vi "Output_SM.vi"(0 "SM Private Data in":refnum<class "Inspection Statemachine.lvclass">, 5 "Output Cluster":T1={"RackID"=0, "Trigger Light Camera Sequence"={"Light Sequence Trigger"="", "Status"="", "Mode"=""}, "Result Cluster"={"RackID"=0, "MeasurementValuesArray "=[], "ImagesArray"=[], "ResultPF"=FALSE, "ProductionCountDetails"={"TotalFail"=0, "TotalPass"=0, "TotalCount"=0}, "ReelCountDetails"={"ReelFail"=0, "ReelPass"=0, "ReelCount"=0}, "ControlPFArray"=[], "SpecificationPFArray"=[], "SpecificationFail"=FALSE, "ReelNumber"=0, "Status"=""}, "Analytics VI refnum"=refnum, "Statistical parameters "=[], "Sensor Name"="", "Camera Name"="", "PopupInput"={"Pop-up Type"=enum."Open Logo Display", "Title"="", "Message"="", "Button 1 Text"="", "Button 2 Text"="", "Show Close? T/F"=FALSE, "Title Blink? T/F"=FALSE, "Title Blink Colour"=0}, "PartInfo"={"PartName"="", "NumberOfRacks"=0, "TotalCount"=0, "ReelCount"=0, "OperatorName"="", "StampingMachineID"=0, "RackID"=0, "Reinitialize"=FALSE, "MeasurementNamesArray"=[], "MeasurementIDArray"=[], "SpecValuesArray"=[], "CameraNamesArray"=[]}, "StateMsgToMI"="", "InspectionStatusToMI"="", "StateMsgToRC"="", "StateMsgToUI"="", "StateMsgToDL"="", "StateMsgToAN"="", "StateMsgToSM"="", "EventData"={"EventName"="", "EventReason"=""}, "CameraOpticsDiagnosticsResult"={"LightCameraName"="", "DiagnosedImage"=refnum, "DustPercentage"=0.0, "Result"=TRUE}, "AllPartInfo"=[{"PartName"="", "NumberOfRacks"=0, "MeasurementIDsArray"=[], "MeasurementNamesArray"=[], "SpecValuesArray"=[]}], "SystemParameters"={"SystemName"="", "SystemID"="", "CustomerDetails"={"CustomerName"="", "CustomerId"="", "Location"="", "NumberOfShifts"=0.0, "ShiftDetails"=[]}, "InstallationDate"="", "NextServiceDate"="", "NumberOfRacks"=0, "TotalNumberOfCameras"=0, "SoftwareFeatures"={"HardwareEmulated"=FALSE, "PowerOnSelfTest"=FALSE, "DiagnosticsEnable"=FALSE, "AnalyticsEnable"=FALSE, "DefectTrackingEnable"=FALSE, "AutomaticGuideMovement"=FALSE, "DoorPokayokeEnable"=FALSE, "FailCountDisplayEnable"=FALSE, "FailCountReversalEnable"=FALSE, "DataLoggingEnable"=FALSE, "PauseOnReelCountFinish"=FALSE, "StopOnTotalCountFinish"=FALSE, "IoTEnable"=FALSE, "ReportEnable"=FALSE, "DebugLevel"=0.0, "PowerOnSelfTestFeatures"={"TimingUnit"=FALSE, "MachinePowerStatusCheck"=FALSE, "GuideMotor"=FALSE, "CameraOptics"=FALSE, "MasterSample"=FALSE}, "DiagnosticsFeatures"={"TimingUnit"=FALSE, "GuideMotor"=FALSE, "CameraOptics"=FALSE, "ReelerMotor"=FALSE, "HardwareButtons"=FALSE, "Sensors"=FALSE, "TowerLamp"=FALSE, "MasterSample"=FALSE}, "UserInterface"={"DynamicImageHandlingEnable"=FALSE, "DoorPokaYokeButtonVisible"=FALSE, "FailCountDisplayButtonVisible"=FALSE, "FailCountReversalButtonVisible"=FALSE}, "PopupOptions"={"ReasonForPause"=FALSE, "ReasonForFail"=FALSE, "ReasonForStop"=FALSE, "CpCpkOnReelFinish"=FALSE}, "DataloggingFeatures"={"EventData"=FALSE, "MeasurementData"=FALSE, "StatisticalData"=FALSE, "ReelData"=FALSE, "FailedMeasurementData"=FALSE, "FailedImages"=FALSE}, "IoT"={"SMSAlertEnable"=FALSE, "EmailAlertEnable"=FALSE}}}, "PartsConfigured"=[], "CameraSequenceList"=[], "SensorList"=[], "MasterSampleMessages"={"MasterSampleMessage"="", "PartMessage"=""}, "SensorDiagnosticsResult"={"Image Array"=[], "ImageCount"=0}, "IgnoredCountDetails"={"ReelCount"=0, "TotalCount"=0}, "MachineStatusToDL"="", "MasterSamplePartName"=""}, 7 "Receiver Name":string(combo), 9 "State":string, 11 "error in (no error)":errorcluster) -> (4 "SM Private Data out":refnum<class "Inspection Statemachine.lvclass">, 15 "error out":errorcluster)   [LabVIEW 2019, in "Inspection Statemachine.lvclass"]
uses:
  Inspection Statemachine.lvclass
  Rack Controller/Rack Controller Messages/RackId_RC Msg/Rack ID_RC Msg.lvclass
  Machine Interface/Machine Interface Messages/State Message from Inspection StateMachine Msg/State Message from Inspection StateMachine Msg_MI.lvclass
  Machine Interface/Machine Interface Messages/Trigger Light Camera Sequence Msg/Trigger Light Camera Sequence Msg_MI.lvclass
  Machine Interface/Machine Interface Messages/Enable and Power On sensor Msg/Enable and Power On Sensor_MI Msg.lvclass
  Machine Interface/Machine Interface Messages/Part Name from Inspection Statemachine Msg/Part Name from Inspection Statemachine Msg_MI.lvclass
  Machine Interface/Machine Interface Messages/Inspection Status Msg/Inspection Status Msg_MI.lvclass
  Rack Controller/Rack Controller Messages/StateMessage_RC Msg/State Message_RC Msg.lvclass
  Rack Controller/Rack Controller Messages/CameraOpticsDiagnostics_RC Msg/Camera Optics Diagnostics_RC Msg.lvclass
  Rack Controller/Rack Controller Messages/Selected Part Info_RC Msg/Selected Part Info_RC Msg.lvclass
  <vilib>/ActorFramework/Actor/Actor.lvclass
  <vilib>/ActorFramework/Message Enqueuer/Message Enqueuer.lvclass
  User Interface/User Interface Messages/User Interface messages/Pre-select init_UI Msg/SystemInfo_UI.lvclass
  User Interface/User Interface Actor/Type Definitions/JSON Read/Data initialization.ctl
  User Interface/User Interface Actor/ZenGage v3.0 UI.lvclass
  User Interface/User Interface Messages/User Interface messages/AN_Get analytics VI ref_UI Msg/GetAnalyticsVI_UI.lvclass
  DataLogger/DataLogger Messages/Part based Initialization_DL Msg/Part based Initialization_DL Msg.lvclass
  DataLogger/DataLogger Messages/Reel Info_DL Msg/Reel Info_DL Msg.lvclass
  DataLogger/DataLogger Messages/Event Info_DL Msg/Event Info_DL Msg.lvclass
  <vilib>/vision/Image Controls.llb/IMAQ Image.ctl
  DataLogger/DataLogger Messages/Statistical Info_DL Msg/Statistical Info_DL Msg.lvclass
  DataLogger/DataLogger Messages/Batch Info_DL Msg/Batch Info_DL Msg.lvclass
  DataLogger/DataLogger Messages/State Message_DL Msg/State Message_DL Msg.lvclass
  DataLogger/DataLogger Messages/AllPartInitialization_DL Msg/AllPartInitialization_DL Msg.lvclass
  DataLogger/DataLogger Messages/System Info_DL Msg/System Info_DL Msg.lvclass
  User Interface/User Interface Messages/User Interface messages/Display Popup Msg/DisplayPopup_UI.lvclass
  User Interface/User Interface Messages/User Interface messages/Call function_UI Msg/ButtonPress_UI.lvclass
  User Interface/User Interface Messages/User Interface messages/Post-select init_UI Msg/PartInfo_UI.lvclass
  User Interface/User Interface Actor/Type Definitions/JSON Read/Post select init.ctl
  User Interface/User Interface Messages/User Interface messages/RC_Result Cluster User Event_UI Msg/DisplayResult_UI Msg.lvclass
  User Interface/User Interface Actor/Type Definitions/Inspection/Result Cluster.ctl
  User Interface/User Interface Messages/User Interface messages/AskEventReason_UI Msg/AskEventReason_UI Msg.lvclass
  ZenAnalytics/Zen Analytics Messages/InterDataCommunication_ZA Msg/InterDataCommunication_ZA Msg.lvclass
  User Interface/User Interface Messages/User Interface messages/Display CpCpk data_UI Msg/Display CpCpk data_UI Msg.lvclass
  Common/Controls/Camera Optics Diagnostics.ctl
  User Interface/User Interface Messages/User Interface messages/Display master sample messages_UI Msg/DisplayMasterSampleMessages_UI Msg.lvclass
  User Interface/User Interface Messages/User Interface messages/CC_Sensor Trigger_UI Msg/TriggerSensorDiagnostics_UI.lvclass
  User Interface/User Interface Messages/User Interface messages/CC_Optics User Event_UI Msg/OpticsDiagnostics_UI.lvclass
  User Interface/User Interface Actor/Type Definitions/User Events UI/Optics diagnostics cluster.ctl
  Inspection Statemachine Messages/ButtonPressed_SM Msg/ButtonPressed_SM Msg.lvclass
  Inspection Statemachine Messages/DiagnosticsResult_SM Msg/DiagnosticsResult_SM Msg.lvclass
  Common/Controls/Diagnostics Result.ctl
  Rack Controller/Rack Controller Messages/IgnoredFailCountDetails_RC Msg/IgnoredFailCountDetails_RC Msg.lvclass
  DataLogger/DataLogger Messages/Measurement Info_DL Msg/Measurement Info_DL Msg.lvclass
  DataLogger/DataLogger Messages/Failure Info_DL Msg/Failure Info_DL Msg.lvclass
  DataLogger/DataLogger Messages/Machine Status_DL Msg/Machine Status_DL Msg.lvclass
  DataLogger/DataLogger Messages/MasterSample Info_DL Msg/MasterSample Info_DL Msg.lvclass
  C:/Program Files/National Instruments/LabVIEW 2019/vi.lib/ActorFramework/Actor/Actor.lvclass
  Controls/Result Cluster_SM.ctl
  Common/Controls/Pop-up Input.ctl
  Controls/Output Cluster_SM.ctl
  Common/Controls/Camera Optics Diagnostics Result.ctl
  Common/Controls/AllPartInfo.ctl
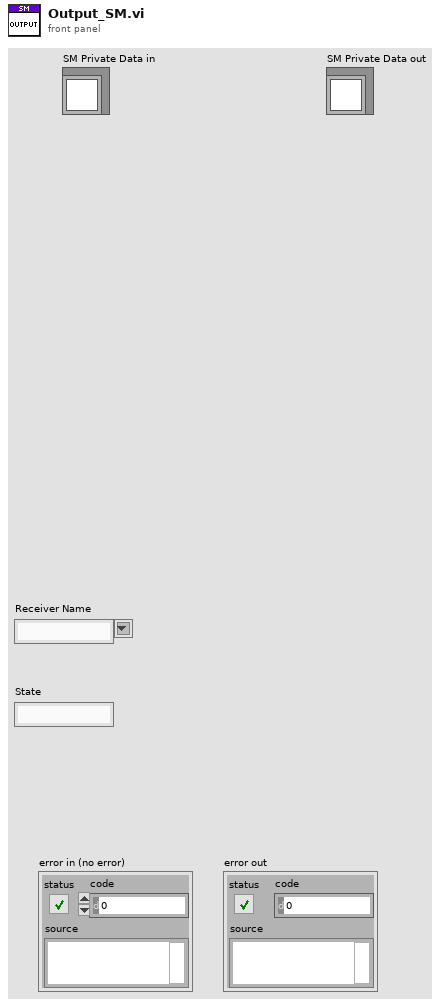
[diagram p1: front panel]
types:
  T1 = typedef "Inspection Statemachine.lvclass/Output Cluster_SM.ctl" = cluster{"RackID":u8, "Trigger Light Camera Sequence":cluster{"Light Sequence Trigger":string, "Status":string, "Mode":string}, "Result Cluster":T2, "Analytics VI refnum":refnum<vi>, "Statistical parameters ":string[][], "Sensor Name":string, "Camera Name":string, "PopupInput":T4, "PartInfo":cluster{"PartName":string, "NumberOfRacks":u8, "TotalCount":u64, "ReelCount":u64, "OperatorName":string, "StampingMachineID":u32, "RackID":u8, "Reinitialize":bool, "MeasurementNamesArray":string[], "MeasurementIDArray":u16[], "SpecValuesArray":cluster{"LCL":dbl, "UCL":dbl, "LSL":dbl, "USL":dbl, "Nominal Value":dbl}[], "CameraNamesArray":string[]}, "StateMsgToMI":string, "InspectionStatusToMI":string, "StateMsgToRC":string, "StateMsgToUI":string, "StateMsgToDL":string, "StateMsgToAN":string, "StateMsgToSM":string, "EventData":cluster{"EventName":string, "EventReason":string}, "CameraOpticsDiagnosticsResult":T5, "AllPartInfo":T6, "SystemParameters":cluster{"SystemName":string, "SystemID":string, "CustomerDetails":cluster{"CustomerName":string, "CustomerId":string, "Location":string, "NumberOfShifts":dbl, "ShiftDetails":cluster{"Name":string, "Timing":string}[]}, "InstallationDate":string, "NextServiceDate":string, "NumberOfRacks":u8, "TotalNumberOfCameras":u8, "SoftwareFeatures":cluster{"HardwareEmulated":bool, "PowerOnSelfTest":bool, "DiagnosticsEnable":bool, "AnalyticsEnable":bool, "DefectTrackingEnable":bool, "AutomaticGuideMovement":bool, "DoorPokayokeEnable":bool, "FailCountDisplayEnable":bool, "FailCountReversalEnable":bool, "DataLoggingEnable":bool, "PauseOnReelCountFinish":bool, "StopOnTotalCountFinish":bool, "IoTEnable":bool, "ReportEnable":bool, "DebugLevel":dbl, "PowerOnSelfTestFeatures":cluster{"TimingUnit":bool, "MachinePowerStatusCheck":bool, "GuideMotor":bool, "CameraOptics":bool, "MasterSample":bool}, "DiagnosticsFeatures":cluster{"TimingUnit":bool, "GuideMotor":bool, "CameraOptics":bool, "ReelerMotor":bool, "HardwareButtons":bool, "Sensors":bool, "TowerLamp":bool, "MasterSample":bool}, "UserInterface":cluster{"DynamicImageHandlingEnable":bool, "DoorPokaYokeButtonVisible":bool, "FailCountDisplayButtonVisible":bool, "FailCountReversalButtonVisible":bool}, "PopupOptions":cluster{"ReasonForPause":bool, "ReasonForFail":bool, "ReasonForStop":bool, "CpCpkOnReelFinish":bool}, "DataloggingFeatures":cluster{"EventData":bool, "MeasurementData":bool, "StatisticalData":bool, "ReelData":bool, "FailedMeasurementData":bool, "FailedImages":bool}, "IoT":cluster{"SMSAlertEnable":bool, "EmailAlertEnable":bool}}}, "PartsConfigured":cluster{"Name":string, "NumberOfRack":u8}[], "CameraSequenceList":cluster{"Name":string, "RackID":u8}[], "SensorList":cluster{"Name":string, "RackID":u8}[], "MasterSampleMessages":cluster{"MasterSampleMessage":string, "PartMessage":string}, "SensorDiagnosticsResult":cluster{"Image Array":T3[], "ImageCount":u64}, "IgnoredCountDetails":cluster{"ReelCount":u64, "TotalCount":u64}, "MachineStatusToDL":string, "MasterSamplePartName":string}
  T2 = typedef "Inspection Statemachine.lvclass/Result Cluster_SM.ctl" = cluster{"RackID":u8, "MeasurementValuesArray ":dbl[], "ImagesArray":T3[], "ResultPF":bool, "ProductionCountDetails":cluster{"TotalFail":u64, "TotalPass":u64, "TotalCount":u64}, "ReelCountDetails":cluster{"ReelFail":u64, "ReelPass":u64, "ReelCount":u64}, "ControlPFArray":bool[], "SpecificationPFArray":bool[], "SpecificationFail":bool, "ReelNumber":u64, "Status":string}
  T3 = typedef "IMAQ Image.ctl" = refnum<image>
  T4 = typedef "Pop-up Input.ctl" = cluster{"Pop-up Type":enum16{"Open Logo Display", "Close Logo Display", "Open Loading Bar", "Close Loading Bar", "Open Alert Display", "Close Alert Display", "One button dialog box", "Two button dialog box", "User Authentication"}, "Title":string, "Message":string, "Button 1 Text":string, "Button 2 Text":string, "Show Close? T/F":bool, "Title Blink? T/F":bool, "Title Blink Colour":u32}
  T5 = typedef "Camera Optics Diagnostics Result.ctl" = cluster{"LightCameraName":string, "DiagnosedImage":T3, "DustPercentage":dbl, "Result":bool}
  T6 = typedef "AllPartInfo.ctl" = cluster{"PartName":string, "NumberOfRacks":u8, "MeasurementIDsArray":u16[], "MeasurementNamesArray":string[], "SpecValuesArray":cluster{"LCL":dbl, "UCL":dbl, "LSL":dbl, "USL":dbl, "NominalValue":dbl}[]}[]
  T7 = typedef "Diagnostics Result.ctl" = cluster{"Result":bool, "StateMessage":string}
  T8 = typedef "Camera Optics Diagnostics.ctl" = cluster{"Light Camera Name":string, " State":string}
  T9 = cluster{"Master sample message":string, "Part message":string}
  T10 = typedef "ZenGage v3.0 UI.lvclass/Post select init.ctl" = cluster{"PartName":string, "RackId":u8, "ReInitialize":bool, "MeasurementNames":string[], "SpecValues":cluster{"LCL":dbl, "UCL":dbl, "LSL":dbl, "USL":dbl, "NominalValue":dbl}[], "CameraNames":string[]}
  T11 = typedef "ZenGage v3.0 UI.lvclass/Data initialization.ctl" = cluster{"DiagnosticsFeatures":cluster{"ArduinoDiagnostics":bool, "MotorDiagnostics":bool, "CameraOpticsDiagnostics":bool, "ReelerMotor":bool, "TowerLampDiagnostics":bool, "HardwareButtonDiagnostics":bool, "TriggerSensor":bool, "MasterSampleDiagnostics":bool}, "UserInterfaceButtonVisibilty":cluster{"Door Poka Yoke":bool, "DynamicImageHandlingEnable":bool, "FailCountDisplayButtonVisible":bool, "FailCountReversalButtonVisible":bool}, "Analytics enabled":bool, "Parts List":cluster{"Part name":string, "NumberOfRacks":u8}[]}
  T12 = cluster{"Reel Count":dbl, "Reel Pass":dbl, "Reel Fail":dbl}
  T13 = cluster{"Total Count":dbl, "Total Pass":dbl, "Total Fail":dbl}
  T14 = typedef "ZenGage v3.0 UI.lvclass/Result Cluster.ctl" = cluster{"Rack Id":u64, "Measurement Values Array ":dbl[], "Images_Array_in":T3[], "ResultPF":bool, "Production count details":cluster{"Total Count":dbl, "Total Pass":dbl, "Total Fail":dbl}, "Control Pass Fail":bool[], "ReelCount Details":cluster{"Reel Count":dbl, "Reel Pass":dbl, "Reel Fail":dbl}, "Specification Pass Fail":bool[], "SpecificationFail":bool}
  T15 = typedef "ZenGage v3.0 UI.lvclass/Optics diagnostics cluster.ctl" = cluster{"DustPercentage":dbl, "Pass":bool, "FinalImage":T3}
  T16 = cluster{"Terminal Count":u32, "isPass":bool, "Terminal Data 1D":dbl[], "Defect":bool[]}
  T17 = cluster{"InitializationParams":cluster{"CurrentPartNumber":string, "Re-Initialize?":bool, "MeasurementData":cluster{"Measurement ID":i32, "Measurement Name":string, "Nominal Values":dbl, "LSL":dbl, "USL":dbl, "LCL":dbl, "UCL":dbl}[]}}
  T18 = cluster{"Measurement ID":i32, "Measurement Name":string, "Nominal Values":dbl, "LSL":dbl, "USL":dbl, "LCL":dbl, "UCL":dbl}
  T19 = cluster{"Part Name":string, "Rack ID":u8, "Reinitialize?":bool, "StampingMc No":u64, "Operator Name":string, "ReelCount":u64, "TotalCount":u64, "Measurement Names Array":string[], "Measurement ID Array":u16[], "Spec Values Array":cluster{"LCL":dbl, "UCL":dbl, "LSL":dbl, "USL":dbl, "Nominal Value":dbl}[], "Camera Name Array":string[]}
  T20 = cluster{"Reel No":u64, "Reel Start Time Stamp":u64}
  T21 = cluster{"FailTimeStamp":u64, "ControlPFArray":bool[], "SpecificationPFArray":dbl[], "FailedImageArray":T3[], "RackID":u8, "Fail Date":string, "Fail Time":string, "Fail Reason":string}
  T22 = cluster{"Statistical Info Array":string[][], "Rack ID":u8}
  T23 = cluster{"Batch Pass Count":u64, "Batch Fail Count":u64, "Rack ID":u8}
  T24 = cluster{"MeasurementDate":string, "MeasurementTime":string, "MeasurementValueArray":dbl[], "MeasurementResult":string}
  T25 = cluster{"System Name":string, "System ID":string, "Version":string, "Year":string, "Customer Details":cluster{"Customer Name":string, "Customer ID":string, "Location":string, "No of Shifts":u8, "Shift Details Array":cluster{"Name":string, "Timing":string}[]}, "Software Features":cluster{"IoT Enable":bool, "Datalogging Features":cluster{"Event Data":bool, "Measurement Data":bool, "Reel Data":bool, "Failed Measurement Data":bool, "Failed Images":bool, bool}, "IoT":cluster{"SMS Alert Enable":bool, "Email Alert Enable":bool}, "Popup Enable?":cluster{"Fail":bool, "Pause":bool, "Stop":bool}}}
  T26 = cluster{"MSPartName":string, "MSDate":string, "MSTime":string, "MSMeasurementValueArray":dbl[], "MSResult":string}
  T27 = cluster{"Light Sequence Trigger":string, "Status":string, "Mode":string}
  T28 = cluster{"PartName":string, "TotalCount":u64, "ReelCount":u64}
  T29 = cluster{"LCL":dbl, "UCL":dbl, "LSL":dbl, "USL":dbl, "Nominal Value":dbl}[]
  T30 = cluster{"TotalFail":u64, "TotalPass":u64, "TotalCount":u64}
  T31 = cluster{"ReelFail":u64, "ReelPass":u64, "ReelCount":u64}
  T32 = cluster{"EventName":string, "date/time string":string, "EventReason":string}
  T33 = cluster{"CustomerName":string, "CustomerId":string, "Location":string, "NumberOfShifts":dbl, "ShiftDetails":cluster{"Name":string, "Timing":string}[]}
  T34 = cluster{"EventData":bool, "MeasurementData":bool, "StatisticalData":bool, "ReelData":bool, "FailedMeasurementData":bool, "FailedImages":bool}
  T35 = cluster{"SMSAlertEnable":bool, "EmailAlertEnable":bool}
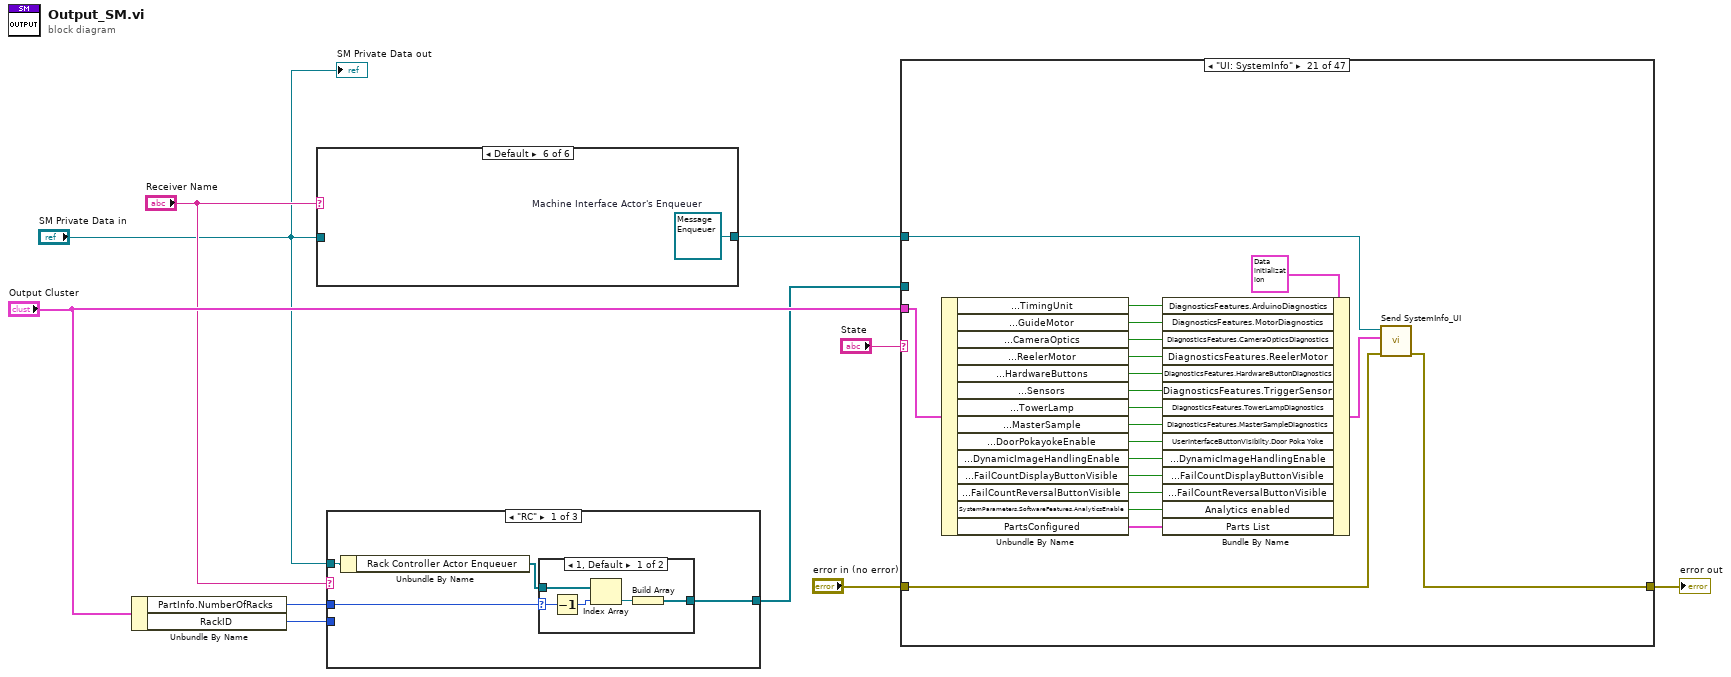
[diagram p0: block diagram]
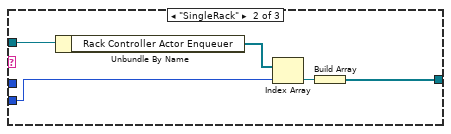
[diagram p3: hidden frame]
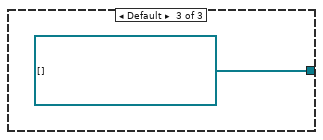
[diagram p4: hidden frame]
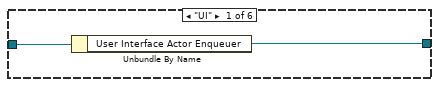
[diagram p5: hidden frame]
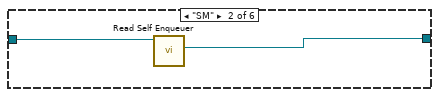
[diagram p6: hidden frame]
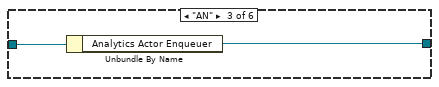
[diagram p7: hidden frame]
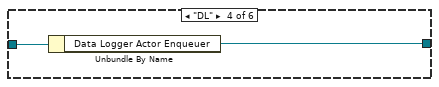
[diagram p8: hidden frame]
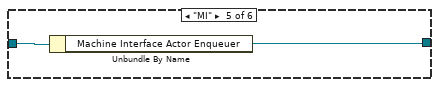
[diagram p9: hidden frame]
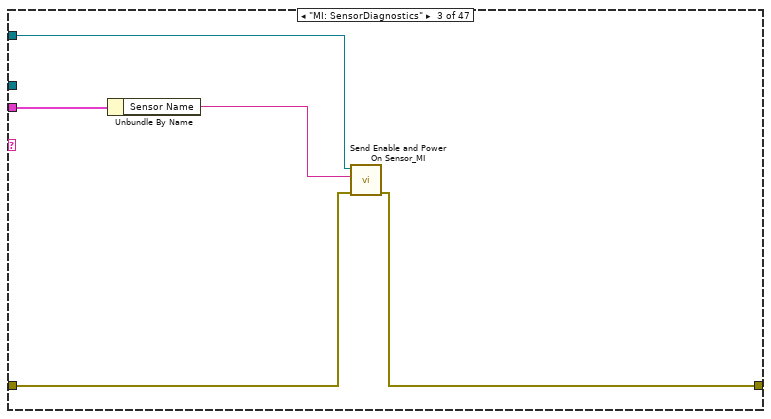
[diagram p12: hidden frame]
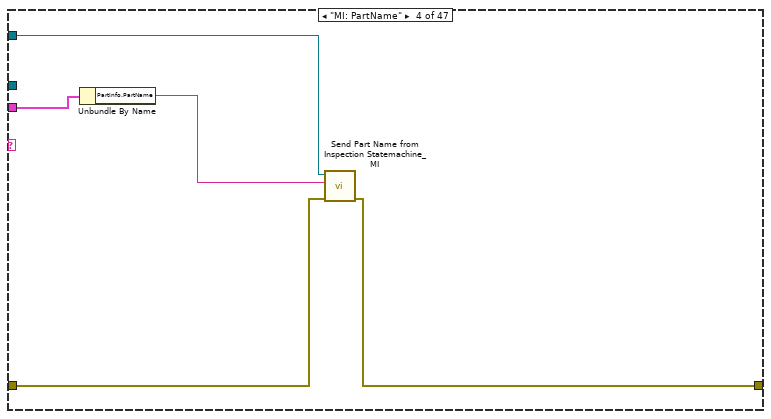
[diagram p13: hidden frame]
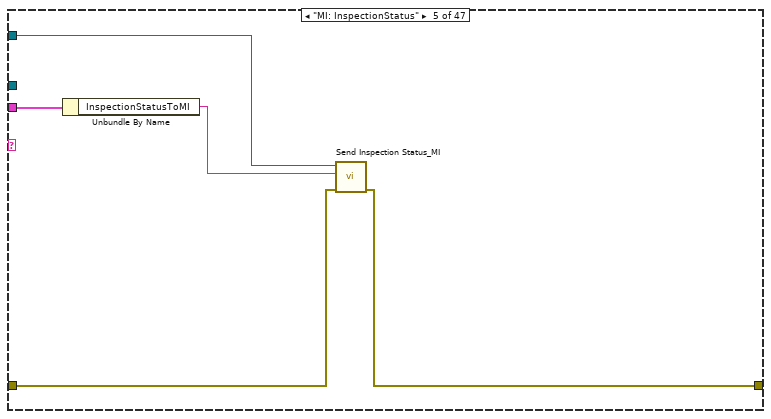
[diagram p14: hidden frame]
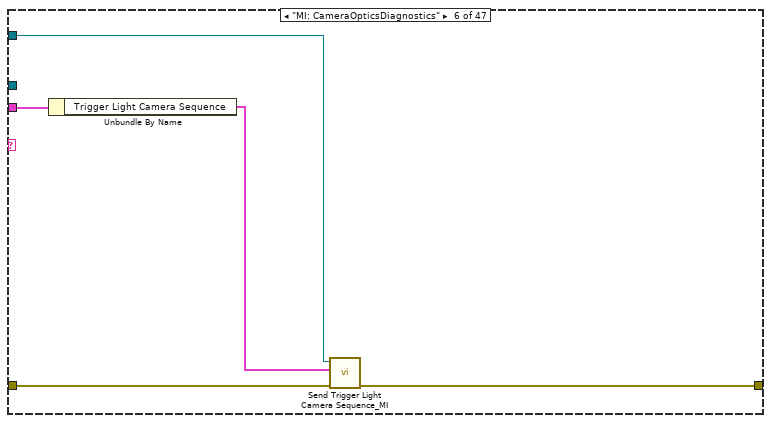
[diagram p15: hidden frame]
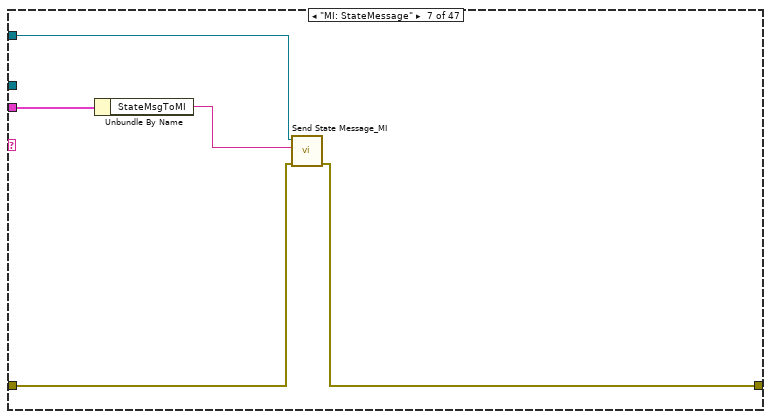
[diagram p16: hidden frame]
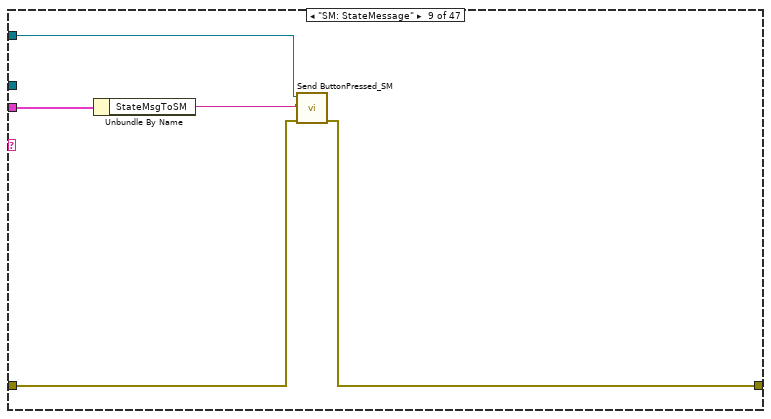
[diagram p18: hidden frame]
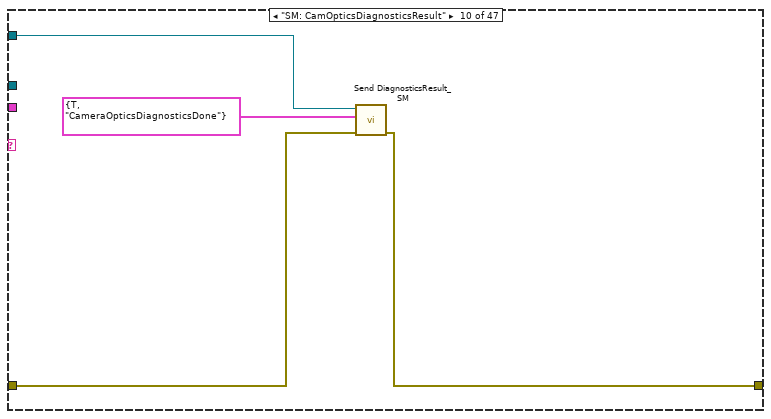
[diagram p19: hidden frame]
diagram:
  n1 = Unbundle By Name("Output Cluster") -> ("PartInfo.NumberOfRacks"=w6:u8, "RackID"=w1:u8)
  n2 = case shown="Default" "Receiver Name" {
    tunnel: "SM Private Data in" -> [w12 w14 w16 w18 w20 _]
    tunnel: [w11 w13 w15 w17 w19 w21] -> w3
    frame "UI" {
      n3 = Unbundle By Name(w12) -> ("User Interface Actor Enqueuer"=w11:refnum<class "Message Enqueuer.lvclass">)
    }
    frame "SM" {
      n4 = call <vilib>:"Read Self Enqueuer.vi"("Actor"=w14) -> ("Self Enqueuer"=w13:refnum<class "Message Enqueuer.lvclass">)  [unwired: 10 in]
    }
    frame "AN" {
      n5 = Unbundle By Name(w16) -> ("Analytics Actor Enqueuer"=w15:refnum<class "Message Enqueuer.lvclass">)
    }
    frame "DL" {
      n6 = Unbundle By Name(w18) -> ("Data Logger Actor Enqueuer"=w17:refnum<class "Message Enqueuer.lvclass">)
    }
    frame "MI" {
      n7 = Unbundle By Name(w20) -> ("Machine Interface Actor Enqueuer"=w19:refnum<class "Message Enqueuer.lvclass">)
    }
    frame Default {
      w21 = refnum<class "Message Enqueuer.lvclass"> refnum  # Machine Interface Actor's Enqueuer
    }
  }
  n8 = case shown="\"RC\"" "Receiver Name" {
    tunnel: "SM Private Data in" -> [w24 w35 _]
    tunnel: w6 -> [w23 _ _]
    tunnel: [w22 w34 refnum<class "Message Enqueuer.lvclass">[] [] ("Rack Controller's Enqueuer")] -> w4
    tunnel: w1 -> [_ w32 _]
    frame "RC" {
      n9 = Unbundle By Name(w24) -> ("Rack Controller Actor Enqueuer"=w25:refnum<class "Message Enqueuer.lvclass">[])
      n10 = case shown="1, Default" w23 {
        selector: w23 -> [w29 _]
        tunnel: [w26 w31] -> w22
        tunnel: w25 -> [w27 w31]
        frame 1, Default {
          n11 = Decrement(x=w29) -> (x-1=w30:u8)
          n12 = Index Array(array=w27, index=w30) -> (element=w28:refnum<class "Message Enqueuer.lvclass">)
          n13 = Build Array(w28) -> (w26:refnum<class "Message Enqueuer.lvclass">[])
        }
        frame 2 {
        }
      }
    }
    frame "SingleRack" {
      n14 = Unbundle By Name(w35) -> ("Rack Controller Actor Enqueuer"=w36:refnum<class "Message Enqueuer.lvclass">[])
      n15 = Index Array(array=w36, index=w32) -> (element=w33:refnum<class "Message Enqueuer.lvclass">)
      n16 = Build Array(w33) -> (w34:refnum<class "Message Enqueuer.lvclass">[])
    }
    frame Default {
    }
  }
  n17 = case shown="\"UI: SystemInfo\"" "State" {
    tunnel: [w38 w39 w41 w48 w53 w58 w62 w65 w68 w73 w75 w77 w83 w97 w107 w119 w125 w127 w134 w140 w169 w185 w196 w202 w211 w215 w222 w226 w229 w231 w240 w253 w261 w270 w295 w310 w315 w323 w341 w357 w365 w382 w387 w392 w410 w415 w432] -> w10
    tunnel: "error in (no error)" -> [w38 w39 w42 w49 w54 w59 w63 w65 w69 w74 w75 w78 w84 w98 w108 w120 w125 w128 w135 w141 w170 w187 w197 w203 w212 w216 w223 w227 w229 w232 w241 w254 w262 w271 w295 w311 w316 w324 w342 w358 w366 w383 w388 w393 w411 w416 w433]
    tunnel: w4 -> [_ _ _ _ _ _ _ _ _ _ _ w76 w86 w99 w104 w113 _ _ _ _ _ _ _ _ _ _ _ _ _ _ _ _ _ _ _ _ _ _ _ _ _ _ _ _ _ _ _]
    tunnel: "Output Cluster" -> [_ _ w44 w47 w52 w56 w64 _ w70 _ _ _ w87 w96 w106 w118 _ w130 w138 w150 w167 w192 w199 w204 w213 w218 w220 w225 _ _ w252 _ _ w284 _ w312 w318 w331 w350 w355 w364 w381 w386 w391 w406 w414 w431]
    tunnel: w3 -> [_ _ w40 w45 w50 w57 w61 _ w66 w72 _ _ _ _ _ _ _ w126 w131 w139 w168 w186 w198 w201 w208 w214 w221 w228 _ w230 w239 w255 w263 w269 _ w298 w320 w322 w343 w356 w367 w384 w389 w394 w409 w413 w434]
    frame Default {
    }
    frame "----------MI----------" {
    }
    frame "MI: SensorDiagnostics" {
      n18 = Unbundle By Name(w44) -> ("Sensor Name"=w43:string)
      n19 = call "Send Enable and Power On Sensor_MI.vi"("error in (no error)"=w42, "Sensor name"=w43, "Message Enqueuer"=w40) -> ("error out"=w41:errorcluster)  [unwired: 7 in, 1 out]
    }
    frame "MI: PartName" {
      n20 = Unbundle By Name(w47) -> ("PartInfo.PartName"=w46:string)
      n21 = call "Send Part Name from Inspection Statemachine_MI.vi"("error in (no error)"=w49, "Part Name"=w46, "Message Enqueuer"=w45) -> ("error out"=w48:errorcluster)  [unwired: 7 in, 1 out]
    }
    frame "MI: InspectionStatus" {
      n22 = Unbundle By Name(w52) -> ("InspectionStatusToMI"=w51:string)
      n23 = call "Send Inspection Status_MI.vi"("error in (no error)"=w54, "Inspection Status"=w51, "Message Enqueuer"=w50) -> ("error out"=w53:errorcluster)  [unwired: 7 in, 1 out]
    }
    frame "MI: CameraOpticsDiagnostics" {
      n24 = Unbundle By Name(w56) -> ("Trigger Light Camera Sequence"=w55:T27)
      n25 = call "Send Trigger Light Camera Sequence_MI.vi"("error in (no error)"=w59, "Trigger Light Camera Sequence"=w55, "Message Enqueuer"=w57) -> ("error out"=w58:errorcluster)  [unwired: 7 in, 1 out]
    }
    frame "MI: StateMessage" {
      n26 = Unbundle By Name(w64) -> ("StateMsgToMI"=w60:string)
      n27 = call "Send State Message_MI.vi"("error in (no error)"=w63, "State Message from Inspection Statemachine"=w60, "Message Enqueuer"=w61) -> ("error out"=w62:errorcluster)  [unwired: 7 in, 1 out]
    }
    frame "----------SM----------" {
    }
    frame "SM: StateMessage" {
      n28 = Unbundle By Name(w70) -> ("StateMsgToSM"=w67:string)
      n29 = call "Send ButtonPressed_SM.vi"("error in (no error)"=w69, "ButtonPress"=w67, "Message Enqueuer"=w66) -> ("error out"=w68:errorcluster)  [unwired: 7 in, 1 out]
    }
    frame "SM: CamOpticsDiagnosticsResult" {
      n30 = call "Send DiagnosticsResult_SM.vi"("error in (no error)"=w74, "DiagnosticsResult"=T7 {"Result"=TRUE, "StateMessage"="CameraOpticsDiagnosticsDone"}, "Message Enqueuer"=w72) -> ("error out"=w73:errorcluster)  [unwired: 7 in, 1 out]
    }
    frame "----------RC----------" {
    }
    frame "RC: RackID" {
      n31 = for {
        shift-right: [w81] -> w77
        shift-left: w78 -> [w82]
        tunnel: w76 -> [w80] mode=indexing
        i -> [w79]
        n32 = call "Send Rack ID_RC.vi"("error in (no error)"=w82, "RackId"=w79, "Message Enqueuer"=w80) -> ("error out"=w81:errorcluster)  [unwired: 7 in, 1 out]
      }
    }
    frame "RC: IgnoredCountDetails" {
      n33 = Unbundle By Name(w87) -> ("IgnoredCountDetails"=w85:cluster{"ReelCount":u64, "TotalCount":u64})
      n34 = for {
        tunnel: w86 -> [w91] mode=indexing
        tunnel: w85 -> [w90]
        shift-right: [w88] -> w83
        shift-left: w84 -> [w89]
        n35 = call "Send IgnoredFailCountDetails_RC.vi"("error in (no error)"=w89, "IgnoredCountDetails"=w90, "Message Enqueuer"=w91) -> ("error out"=w88:errorcluster)  [unwired: 7 in, 1 out]
      }
    }
    frame "RC: CameraOpticsDiagnostics" {
      n36 = Unbundle By Name(w96) -> ("Trigger Light Camera Sequence.Light Sequence Trigger"=w93:string, "Trigger Light Camera Sequence.Status"=w94:string)
      n37 = Bundle By Name(cluster=T8 {"Light Camera Name"="", " State"=""} ("Light Camera Info"), "Light Camera Name"=w93, "State"=w94) -> (w92:T8)
      n38 = for {
        tunnel: w98 -> [w103]
        tunnel: w99 -> [w101] mode=indexing
        tunnel: [w102] -> w97
        tunnel: w92 -> [w100]
        # "This loop iterates \"Number of Racks\" times"
        n39 = call "Send Camera Optics Diagnostics_RC.vi"("error in (no error)"=w103, "Light Camera Info"=w100, "Message Enqueuer"=w101) -> ("error out"=w102:errorcluster)  [unwired: 7 in, 1 out]
      }
    }
    frame "RC: StateMessage" {
      n40 = Unbundle By Name(w106) -> ("StateMsgToRC"=w105:string)
      n41 = for {
        tunnel: w105 -> [w110]
        tunnel: w104 -> [w109] mode=indexing
        shift-right: [w111] -> w107
        shift-left: w108 -> [w112]
        n42 = call "Send State Message_RC.vi"("error in (no error)"=w112, "State Message"=w110, "Message Enqueuer"=w109) -> ("error out"=w111:errorcluster)  [unwired: 7 in, 1 out]
      }
    }
    frame "RC: SelectedPartInfo" {
      n43 = Unbundle By Name(w118) -> ("PartInfo.PartName"=w117:string, "PartInfo.TotalCount"=w116:u64, "PartInfo.ReelCount"=w115:u64)
      n44 = Bundle("PartName"=w117, "TotalCount"=w116, "ReelCount"=w115) -> (w114:T28)  [unwired: 1 in]
      n45 = for {
        tunnel: w114 -> [w122]
        shift-right: [w123] -> w119
        shift-left: w120 -> [w124]
        tunnel: w113 -> [w121] mode=indexing
        n46 = call "Send Selected Part Info_RC.vi"("error in (no error)"=w124, "Part Details"=w122, "Message Enqueuer"=w121) -> ("error out"=w123:errorcluster)  [unwired: 7 in, 1 out]
      }
    }
    frame "----------UI----------" {
    }
    frame "UI: StateMessage" {
      n47 = Unbundle By Name(w130) -> ("StateMsgToUI"=w129:string)
      n48 = call "Send ButtonPress_UI.vi"("error in (no error)"=w128, "FunctionalityName"=w129, "Message Enqueuer"=w126) -> ("error out"=w127:errorcluster)  [unwired: 7 in, 1 out]
    }
    frame "UI: MasterSampleMessages" {
      n49 = Unbundle By Name(w138) -> ("MasterSampleMessages.MasterSampleMessage"=w133:string, "MasterSampleMessages.PartMessage"=w132:string)
      n50 = Bundle By Name(cluster=T9 {"Master sample message"="", "Part message"=""} ("Master sample messages"), "Master sample message"=w133, "Part message"=w132) -> (w137:T9)
      n51 = call "Send DisplayMasterSampleMessages_UI.vi"("error in (no error)"=w135, "Master sample messages"=w137, "Message Enqueuer"=w131) -> ("error out"=w134:errorcluster)  [unwired: 7 in, 1 out]
    }
    frame "UI: PartInfo" {
      n52 = Unbundle By Name(w150) -> ("PartInfo.PartName"=w147:string, "PartInfo.RackID"=w146:u8, "PartInfo.Reinitialize"=w145:bool, "PartInfo.MeasurementNamesArray"=w144:string[], "PartInfo.SpecValuesArray"=w143:T29, "PartInfo.CameraNamesArray"=w142:string[])
      n53 = Bundle By Name(cluster=T10 {"PartName"="", "RackId"=0, "ReInitialize"=FALSE, "MeasurementNames"=[], "SpecValues"=[], "CameraNames"=[]} ("PartInfo\ndata"), "PartName"=w147, "RackId"=w146, "ReInitialize"=w145, "MeasurementNames"=w144, "SpecValues"=w143, "CameraNames"=w142) -> (w148:T10)
      n54 = call "Send PartInfo_UI.vi"("error in (no error)"=w141, "PartInfo\ndata"=w148, "Message Enqueuer"=w139) -> ("error out"=w140:errorcluster)  [unwired: 7 in, 1 out]
    }
    frame "UI: SystemInfo" {
      n55 = Unbundle By Name(w167) -> ("SystemParameters.SoftwareFeatures.DiagnosticsFeatures.TimingUnit"=w164:bool, "SystemParameters.SoftwareFeatures.DiagnosticsFeatures.GuideMotor"=w163:bool, "SystemParameters.SoftwareFeatures.DiagnosticsFeatures.CameraOptics"=w162:bool, "SystemParameters.SoftwareFeatures.DiagnosticsFeatures.ReelerMotor"=w161:bool, "SystemParameters.SoftwareFeatures.DiagnosticsFeatures.HardwareButtons"=w160:bool, "SystemParameters.SoftwareFeatures.DiagnosticsFeatures.Sensors"=w159:bool, "SystemParameters.SoftwareFeatures.DiagnosticsFeatures.TowerLamp"=w158:bool, "SystemParameters.SoftwareFeatures.DiagnosticsFeatures.MasterSample"=w157:bool, "SystemParameters.SoftwareFeatures.DoorPokayokeEnable"=w156:bool, "SystemParameters.SoftwareFeatures.UserInterface.DynamicImageHandlingEnable"=w155:bool, "SystemParameters.SoftwareFeatures.UserInterface.FailCountDisplayButtonVisible"=w154:bool, "SystemParameters.SoftwareFeatures.UserInterface.FailCountReversalButtonVisible"=w153:bool, "SystemParameters.SoftwareFeatures.AnalyticsEnable"=w152:bool, "PartsConfigured"=w151:cluster{"Name":string, "NumberOfRack":u8}[])
      n56 = Bundle By Name(cluster=T11 {"DiagnosticsFeatures"={"ArduinoDiagnostics"=FALSE, "MotorDiagnostics"=FALSE, "CameraOpticsDiagnostics"=FALSE, "ReelerMotor"=FALSE, "TowerLampDiagnostics"=FALSE, "HardwareButtonDiagnostics"=FALSE, "TriggerSensor"=FALSE, "MasterSampleDiagnostics"=FALSE}, "UserInterfaceButtonVisibilty"={"Door Poka Yoke"=FALSE, "DynamicImageHandlingEnable"=FALSE, "FailCountDisplayButtonVisible"=FALSE, "FailCountReversalButtonVisible"=FALSE}, "Analytics enabled"=FALSE, "Parts List"=[]} ("SystemInit\ndata"), "DiagnosticsFeatures.ArduinoDiagnostics"=w164, "DiagnosticsFeatures.MotorDiagnostics"=w163, "DiagnosticsFeatures.CameraOpticsDiagnostics"=w162, "DiagnosticsFeatures.ReelerMotor"=w161, "DiagnosticsFeatures.HardwareButtonDiagnostics"=w160, "DiagnosticsFeatures.TriggerSensor"=w159, "DiagnosticsFeatures.TowerLampDiagnostics"=w158, "DiagnosticsFeatures.MasterSampleDiagnostics"=w157, "UserInterfaceButtonVisibilty.Door Poka Yoke"=w156, "UserInterfaceButtonVisibilty.DynamicImageHandlingEnable"=w155, "UserInterfaceButtonVisibilty.FailCountDisplayButtonVisible"=w154, "UserInterfaceButtonVisibilty.FailCountReversalButtonVisible"=w153, "Analytics enabled"=w152, "Parts List"=w151) -> (w165:T11)
      n57 = call "Send SystemInfo_UI.vi"("error in (no error)"=w170, "SystemInit\ndata"=w165, "Message Enqueuer"=w168) -> ("error out"=w169:errorcluster)  [unwired: 7 in, 1 out]
    }
    frame "UI: ResultData" {
      n58 = Unbundle By Name(w192) -> ("Result Cluster.MeasurementValuesArray"=w191:dbl[], "Result Cluster.ProductionCountDetails"=w182:T30, "Result Cluster.ImagesArray"=w190:T3[], "Result Cluster.ResultPF"=w189:bool, "Result Cluster.ReelCountDetails"=w176:T31, "Result Cluster.ControlPFArray"=w188:bool[], "Result Cluster.SpecificationPFArray"=w184:bool[], "RackID"=w183:u8)
      n59 = Unbundle By Name(w182) -> ("TotalCount"=w180:u64, "TotalPass"=w179:u64, "TotalFail"=w178:u64)
      n60 = Unbundle By Name(w176) -> ("ReelCount"=w174:u64, "ReelPass"=w173:u64, "ReelFail"=w172:u64)
      n61 = Bundle By Name(cluster=T13 {"Total Count"=0.0, "Total Pass"=0.0, "Total Fail"=0.0} ("Production count details"), "Total Count"=w180, "Total Pass"=w179, "Total Fail"=w178) -> (w177:T13)
      n62 = Bundle By Name(cluster=T12 {"Reel Count"=0.0, "Reel Pass"=0.0, "Reel Fail"=0.0} ("ReelCount Details"), "Reel Count"=w174, "Reel Pass"=w173, "Reel Fail"=w172) -> (w171:T12)
      n63 = Bundle By Name(cluster=T14 {"Rack Id"=0, "Measurement Values Array "=[], "Images_Array_in"=[], "ResultPF"=FALSE, "Production count details"={"Total Count"=0.0, "Total Pass"=0.0, "Total Fail"=0.0}, "Control Pass Fail"=[], "ReelCount Details"={"Reel Count"=0.0, "Reel Pass"=0.0, "Reel Fail"=0.0}, "Specification Pass Fail"=[], "SpecificationFail"=FALSE} ("Result Cluster"), "Measurement Values Array"=w191, "Production count details"=w177, "Images_Array_in"=w190, "ResultPF"=w189, "ReelCount Details"=w171, "Control Pass Fail"=w188, "Specification Pass Fail"=w184, "Rack Id"=w183) -> (w193:T14)
      n64 = call "Send DisplayResult_UI.vi"("error in (no error)"=w187, "Result Cluster"=w193, "Message Enqueuer"=w186) -> ("error out"=w185:errorcluster)  [unwired: 7 in, 1 out]
    }
    frame "UI: AskEventReason" {
      n65 = Unbundle By Name(w199) -> ("StateMsgToUI"=w195:string)
      n66 = call "Send AskEventReason_UI.vi"("error in (no error)"=w197, "Event state name"=w195, "Message Enqueuer"=w198) -> ("error out"=w196:errorcluster)  [unwired: 7 in, 1 out]
    }
    frame "UI: DisplayPopup" {
      n67 = Unbundle By Name(w204) -> ("PopupInput"=w200:T4)
      n68 = call "Send DisplayPopup_UI.vi"("error in (no error)"=w203, "PopupDetails"=w200, "Message Enqueuer"=w201) -> ("error out"=w202:errorcluster)  [unwired: 7 in, 1 out]
    }
    frame "UI: CameraOpticsDiagnosticsResult" {
      n69 = Unbundle By Name(w213) -> ("CameraOpticsDiagnosticsResult.DustPercentage"=w207:dbl, "CameraOpticsDiagnosticsResult.Result"=w206:bool, "CameraOpticsDiagnosticsResult.DiagnosedImage"=w205:T3)
      n70 = Bundle By Name(cluster=T15 {"DustPercentage"=90.0, "Pass"=FALSE, "FinalImage"=refnum} ("Optics User Event in"), "DustPercentage"=w207, "Pass"=w206, "FinalImage"=w205) -> (w209:T15)
      n71 = call "Send OpticsDiagnostics_UI.vi"("error in (no error)"=w212, "Optics User Event in"=w209, "Message Enqueuer"=w208) -> ("error out"=w211:errorcluster)  [unwired: 7 in, 1 out]
    }
    frame "UI: SensorDiagnosticsResult" {
      n72 = Unbundle By Name(w218) -> ("SensorDiagnosticsResult"=w217:cluster{"Image Array":T3[], "ImageCount":u64})
      n73 = call "Send TriggerSensorDiagnostics_UI.vi"("error in (no error)"=w216, "Cluster"=w217, "Message Enqueuer"=w214) -> ("error out"=w215:errorcluster)  [unwired: 7 in, 1 out]
    }
    frame "UI: AnalyticsRef" {
      n74 = Unbundle By Name(w220) -> ("Analytics VI refnum"=w219:refnum<vi>)
      n75 = call "Send AnalyticsVIRefnum_UI.vi"("error in (no error)"=w223, "Analytics VI\nrefnum"=w219, "Message Enqueuer"=w221) -> ("error out"=w222:errorcluster)  [unwired: 7 in, 1 out]
    }
    frame "UI: StatisticalParameters" {
      n76 = Unbundle By Name(w225) -> ("Statistical parameters"=w224:string[][])
      n77 = call "Send Display CpCpk data_UI.vi"("error in (no error)"=w227, "event data"=w224, "Message Enqueuer"=w228) -> ("error out"=w226:errorcluster)  [unwired: 7 in, 1 out]
    }
    frame "----------Analytics----------" {
    }
    frame "AN: GetStatisticalparameters" {
      n78 = To Variant(anything=TRUE ("Back")) -> (Variant=w234:variant)
      n79 = Bundle By Name(cluster=cluster{"State Name":string, "Data":variant} {"State Name"="Init", "Data"=variant} ("Inter Actor event data"), "State Name"="StatisticalData", "Data"=w234) -> (w235:cluster{"State Name":string, "Data":variant})
      n80 = call "Send InterDataCommunication_ZA.vi"("error in (no error)"=w232, "InterDataCommunication_ZA"=w235, "Message Enqueuer"=w230) -> ("error out"=w231:errorcluster)  [unwired: 7 in, 1 out]
    }
    frame "AN: ResultData" {
      n81 = Unbundle By Name(w252) -> ("Result Cluster.ReelCountDetails.ReelCount"=w249:u64, "Result Cluster.ResultPF"=w250:bool, "Result Cluster.MeasurementValuesArray"=w248:dbl[], "Result Cluster.ControlPFArray"=w246:bool[])
      n82 = Not(x=w246) -> (.not. x?=w247:bool[])
      n83 = Bundle By Name(cluster=T16 {"Terminal Count"=0, "isPass"=FALSE, "Terminal Data 1D"=[], "Defect"=[]} ("ResultCluster"), "Terminal Count"=w249, "isPass"=w250, "Terminal Data 1D"=w248, "Defect"=w247) -> (w238:T16)
      n84 = To Variant(anything=w238) -> (Variant=w242:variant)
      n85 = Bundle By Name(cluster=cluster{"State Name":string, "Data":variant} {"State Name"="Init", "Data"=variant} ("Inter Actor event data"), "State Name"="ResultData", "Data"=w242) -> (w243:cluster{"State Name":string, "Data":variant})
      n86 = call "Send InterDataCommunication_ZA.vi"("error in (no error)"=w241, "InterDataCommunication_ZA"=w243, "Message Enqueuer"=w239) -> ("error out"=w240:errorcluster)  [unwired: 7 in, 1 out]
    }
    frame "AN: ToAnalytics" {
      n87 = To Variant(anything=TRUE ("Back")) -> (Variant=w257:variant)
      n88 = Bundle By Name(cluster=cluster{"State Name":string, "Data":variant} {"State Name"="Init", "Data"=variant} ("Inter Actor event data"), "State Name"="Analytics", "Data"=w257) -> (w258:cluster{"State Name":string, "Data":variant})
      n89 = call "Send InterDataCommunication_ZA.vi"("error in (no error)"=w254, "InterDataCommunication_ZA"=w258, "Message Enqueuer"=w255) -> ("error out"=w253:errorcluster)  [unwired: 7 in, 1 out]
    }
    frame "AN: ToImages" {
      n90 = To Variant(anything=TRUE ("Back")) -> (Variant=w265:variant)
      n91 = Bundle By Name(cluster=cluster{"State Name":string, "Data":variant} {"State Name"="Init", "Data"=variant} ("Inter Actor event data"), "State Name"="Back", "Data"=w265) -> (w266:cluster{"State Name":string, "Data":variant})
      n92 = call "Send InterDataCommunication_ZA.vi"("error in (no error)"=w262, "InterDataCommunication_ZA"=w266, "Message Enqueuer"=w263) -> ("error out"=w261:errorcluster)  [unwired: 7 in, 1 out]
    }
    frame "AN: PartInfo" {
      n93 = Unbundle By Name(w284) -> ("PartInfo.PartName"=w278:string, "PartInfo.Reinitialize"=w277:bool, "PartInfo.MeasurementIDArray"=w283:u16[], "PartInfo.MeasurementNamesArray"=w282:string[], "PartInfo.SpecValuesArray"=w281:T29)
      n94 = for {
        tunnel: w283 -> [w292] mode=indexing
        tunnel: w282 -> [w291] mode=indexing
        tunnel: w281 -> [w294] mode=indexing
        tunnel: [w285] -> w279 mode=indexing
        n95 = Unbundle By Name(w294) -> ("Nominal Value"=w290:dbl, "LSL"=w289:dbl, "USL"=w288:dbl, "LCL"=w287:dbl, "UCL"=w286:dbl)
        n96 = Bundle By Name(cluster=T18 {"Measurement ID"=0, "Measurement Name"="", "Nominal Values"=0.0, "LSL"=0.0, "USL"=0.0, "LCL"=0.0, "UCL"=0.0}, "Measurement ID"=w292, "Measurement Name"=w291, "Nominal Values"=w290, "LSL"=w289, "USL"=w288, "LCL"=w287, "UCL"=w286) -> (w285:T18)
      }
      n97 = Bundle By Name(cluster=T17 {"InitializationParams"={"CurrentPartNumber"="", "Re-Initialize?"=FALSE, "MeasurementData"=[]}} ("Initialization Values"), "InitializationParams.CurrentPartNumber"=w278, "InitializationParams.Re-Initialize?"=w277, "InitializationParams.MeasurementData"=w279) -> (w272:T17)
      n98 = To Variant(anything=w272) -> (Variant=w273:variant)
      n99 = Bundle By Name(cluster=cluster{"State Name":string, "Data":variant} {"State Name"="Init", "Data"=variant} ("Inter Actor event data"), "State Name"="Init", "Data"=w273) -> (w274:cluster{"State Name":string, "Data":variant})
      n100 = call "Send InterDataCommunication_ZA.vi"("error in (no error)"=w271, "InterDataCommunication_ZA"=w274, "Message Enqueuer"=w269) -> ("error out"=w270:errorcluster)  [unwired: 7 in, 1 out]
    }
    frame "----------DataLogger----------" {
    }
    frame "DL: PartInfo" {
      n101 = Unbundle By Name(w312) -> ("PartInfo.PartName"=w309:string, "PartInfo.RackID"=w308:u8, "PartInfo.Reinitialize"=w307:bool, "PartInfo.StampingMachineID"=w306:u32, "PartInfo.OperatorName"=w305:string, "PartInfo.ReelCount"=w304:u64, "PartInfo.TotalCount"=w303:u64, "PartInfo.MeasurementNamesArray"=w302:string[], "PartInfo.MeasurementIDArray"=w301:u16[], "PartInfo.SpecValuesArray"=w300:T29, "PartInfo.CameraNamesArray"=w299:string[])
      n102 = Bundle By Name(cluster=T19 {"Part Name"="", "Rack ID"=0, "Reinitialize?"=FALSE, "StampingMc No"=0, "Operator Name"="", "ReelCount"=0, "TotalCount"=0, "Measurement Names Array"=[], "Measurement ID Array"=[], "Spec Values Array"=[], "Camera Name Array"=[]} ("Part Info"), "Part Name"=w309, "Rack ID"=w308, "Reinitialize?"=w307, "StampingMc No"=w306, "Operator Name"=w305, "ReelCount"=w304, "TotalCount"=w303, "Measurement Names Array"=w302, "Measurement ID Array"=w301, "Spec Values Array"=w300, "Camera Name Array"=w299) -> (w296:T19)
      n103 = call "Send Part based Initialization_DL.vi"("error in (no error)"=w311, "Part Info"=w296, "Message Enqueuer"=w298) -> ("error out"=w310:errorcluster)  [unwired: 7 in, 1 out]
    }
    frame "DL: ReelInfo" {
      # "Generate a timestamp for reelstart"
      n104 = Unbundle By Name(w318) -> ("Result Cluster.ReelNumber"=w317:u64)
      n105 = Get Date/Time In Seconds() -> (seconds since 1Jan1904=w321:timestamp)
      n106 = To Unsigned Quad Integer(1:w321) -> (0:w319:u64)
      n107 = Bundle By Name(cluster=T20 {"Reel No"=0, "Reel Start Time Stamp"=0} ("Reel Info"), "Reel No"=w317, "Reel Start Time Stamp"=w319) -> (w313:T20)
      n108 = call "Send Reel Info_DL.vi"("error in (no error)"=w316, "Reel Info"=w313, "Message Enqueuer"=w320) -> ("error out"=w315:errorcluster)  [unwired: 7 in, 1 out]
    }
    frame "DL: EventDetails" {
      n109 = Unbundle By Name(w331) -> ("EventData.EventName"=w330:string, "EventData.EventReason"=w329:string)
      n110 = Get Date/Time In Seconds() -> (seconds since 1Jan1904=w328:timestamp)
      n111 = Format Date/Time String(time format string (%c)="%d-%b-%Y %H:%M:%S", seconds (now)=w328) -> (date/time string=w326:string)  [unwired: 1 in]
      n112 = Bundle("EventName"=w330, "date/time string"=w326, "EventReason"=w329) -> (w325:T32)  [unwired: 1 in]
      n113 = call "Send Event Info_DL.vi"("error in (no error)"=w324, "Event Info"=w325, "Message Enqueuer"=w322) -> ("error out"=w323:errorcluster)  [unwired: 7 in, 1 out]
    }
    frame "DL: FailureDetails" {
      # "%d-%b-%Y %H:%M:%S"
      n114 = Get Date/Time In Seconds() -> (seconds since 1Jan1904=w338:timestamp)
      n115 = Get Date/Time In Seconds() -> (seconds since 1Jan1904=w334:timestamp)
      n116 = Unbundle By Name(w350) -> ("Result Cluster.ControlPFArray"=w347:bool[], "Result Cluster.MeasurementValuesArray"=w346:dbl[], "Result Cluster.ImagesArray"=w345:T3[], "EventData.EventReason"=w332:string)
      n117 = Get Date/Time In Seconds() -> (seconds since 1Jan1904=w348:timestamp)
      n118 = Format Date/Time String(time format string (%c)="%d-%b-%Y", seconds (now)=w338) -> (date/time string=w336:string)  [unwired: 1 in]
      n119 = To Unsigned Long Integer(number=w348) -> (unsigned 32bit integer=w344:u32)
      n120 = Format Date/Time String(time format string (%c)="%H:%M", seconds (now)=w334) -> (date/time string=w333:string)  [unwired: 1 in]
      n121 = Bundle By Name(cluster=T21 {"FailTimeStamp"=0, "ControlPFArray"=[], "SpecificationPFArray"=[], "FailedImageArray"=[], "RackID"=0, "Fail Date"="", "Fail Time"="", "Fail Reason"=""} ("Failure Info"), "FailTimeStamp"=w344, "ControlPFArray"=w347, "SpecificationPFArray"=w346, "FailedImageArray"=w345, "RackID"=u8 0, "Fail Date"=w336, "Fail Time"=w333, "Fail Reason"=w332) -> (w339:T21)
      n122 = call "Send Failure Info_DL.vi"("error in (no error)"=w342, "Failure Info"=w339, "Message Enqueuer"=w343) -> ("error out"=w341:errorcluster)  [unwired: 7 in, 1 out]
    }
    frame "DL: StatisticalDetails" {
      # "To be modified."
      n123 = Unbundle By Name(w355) -> ("Statistical parameters"=w351:string[][])
      n124 = Bundle By Name(cluster=T22 {"Statistical Info Array"=[], "Rack ID"=0} ("Statistical Info"), "Statistical Info Array"=w351, "Rack ID"=u8 0) -> (w353:T22)
      n125 = call "Send Statistical Info_DL.vi"("error in (no error)"=w358, "Statistical Info"=w353, "Message Enqueuer"=w356) -> ("error out"=w357:errorcluster)  [unwired: 7 in, 1 out]
    }
    frame "DL: BatchDetails" {
      n126 = Unbundle By Name(w364) -> ("Result Cluster.ReelCountDetails.ReelPass"=w360:u64, "Result Cluster.ReelCountDetails.ReelFail"=w359:u64)
      n127 = Bundle By Name(cluster=T23 {"Batch Pass Count"=0, "Batch Fail Count"=0, "Rack ID"=0} ("Batch Info"), "Batch Pass Count"=w360, "Batch Fail Count"=w359, "Rack ID"=u8 0) -> (w363:T23)
      n128 = call "Send Batch Info_DL.vi"("error in (no error)"=w366, "Batch Info"=w363, "Message Enqueuer"=w367) -> ("error out"=w365:errorcluster)  [unwired: 7 in, 1 out]
    }
    frame "DL: MeasurementDetails" {
      n129 = Unbundle By Name(w381) -> ("Result Cluster.MeasurementValuesArray"=w372:dbl[], "Result Cluster.ResultPF"=w371:bool)
      n130 = Get Date/Time In Seconds() -> (seconds since 1Jan1904=w378:timestamp)
      n131 = Get Date/Time In Seconds() -> (seconds since 1Jan1904=w375:timestamp)
      n132 = Format Date/Time String(time format string (%c)="%d-%b-%Y", seconds (now)=w378) -> (date/time string=w376:string)  [unwired: 1 in]
      n133 = Format Date/Time String(time format string (%c)="%H:%M", seconds (now)=w375) -> (date/time string=w374:string)  [unwired: 1 in]
      n134 = Select(t="Pass", s=w371, f="Fail") -> (s? t:f=w368:string)
      n135 = Bundle By Name(cluster=T24 {"MeasurementDate"="", "MeasurementTime"="", "MeasurementValueArray"=[], "MeasurementResult"=""} ("Measurement Info"), "MeasurementDate"=w376, "MeasurementTime"=w374, "MeasurementValueArray"=w372, "MeasurementResult"=w368) -> (w379:T24)
      n136 = call "Send Measurement Info_DL.vi"("error in (no error)"=w383, "Measurement Info"=w379, "Message Enqueuer"=w384) -> ("error out"=w382:errorcluster)  [unwired: 7 in, 1 out]
    }
    frame "DL: StateMessage" {
      n137 = Unbundle By Name(w386) -> ("StateMsgToDL"=w385:string)
      n138 = call "Send State Message_DL.vi"("error in (no error)"=w388, "State Message"=w385, "Message Enqueuer"=w389) -> ("error out"=w387:errorcluster)  [unwired: 7 in, 1 out]
    }
    frame "DL: MachineStatus" {
      n139 = Unbundle By Name(w391) -> ("MachineStatusToDL"=w390:string)
      n140 = call "Send Machine Status_DL.vi"("error in (no error)"=w393, "MachineStatus"=w390, "Message Enqueuer"=w394) -> ("error out"=w392:errorcluster)  [unwired: 7 in, 1 out]
    }
    frame "DL: SystemInfo" {
      n141 = Unbundle By Name(w406) -> ("SystemParameters.SystemName"=w404:string, "SystemParameters.SystemID"=w403:string, "SystemParameters.CustomerDetails"=w405:T33, "SystemParameters.SoftwareFeatures.IoTEnable"=w402:bool, "SystemParameters.SoftwareFeatures.DataloggingFeatures"=w395:T34, "SystemParameters.SoftwareFeatures.IoT"=w401:T35, "SystemParameters.SoftwareFeatures.PopupOptions.ReasonForFail"=w400:bool, "SystemParameters.SoftwareFeatures.PopupOptions.ReasonForPause"=w399:bool, "SystemParameters.SoftwareFeatures.PopupOptions.ReasonForStop"=w398:bool, "SystemParameters.InstallationDate"=w397:string)
      n142 = Bundle By Name(cluster=T25 {"System Name"="", "System ID"="", "Version"="", "Year"="", "Customer Details"={"Customer Name"="", "Customer ID"="", "Location"="", "No of Shifts"=0, "Shift Details Array"=[]}, "Software Features"={"IoT Enable"=FALSE, "Datalogging Features"={"Event Data"=FALSE, "Measurement Data"=FALSE, "Reel Data"=FALSE, "Failed Measurement Data"=FALSE, "Failed Images"=FALSE, FALSE}, "IoT"={"SMS Alert Enable"=FALSE, "Email Alert Enable"=FALSE}, "Popup Enable?"={"Fail"=FALSE, "Pause"=FALSE, "Stop"=FALSE}}} ("System Info"), "System Name"=w404, "System ID"=w403, "Customer Details"=w405, "Software Features.IoT Enable"=w402, "Software Features.Datalogging Features"=w395, "Software Features.IoT"=w401, "Software Features.Popup Enable?.Fail"=w400, "Software Features.Popup Enable?.Pause"=w399, "Software Features.Popup Enable?.Stop"=w398, "Version"="V1.3", "Year"=w397) -> (w407:T25)
      n143 = call "Send System Info_DL.vi"("error in (no error)"=w411, "System Info"=w407, "Message Enqueuer"=w409) -> ("error out"=w410:errorcluster)  [unwired: 7 in, 1 out]
    }
    frame "DL: AllPartInfo" {
      n144 = Unbundle By Name(w414) -> ("AllPartInfo"=w412:T6)
      n145 = call "Send AllPartInitialization_DL.vi"("error in (no error)"=w416, "AllPartInfoArray"=w412, "Message Enqueuer"=w413) -> ("error out"=w415:errorcluster)  [unwired: 7 in, 1 out]
    }
    frame "DL: MasterSampleDetails" {
      n146 = Unbundle By Name(w431) -> ("Result Cluster.MeasurementValuesArray"=w424:dbl[], "Result Cluster.ResultPF"=w428:bool, "MasterSamplePartName"=w417:string)
      n147 = Get Date/Time In Seconds() -> (seconds since 1Jan1904=w421:timestamp)
      n148 = Get Date/Time In Seconds() -> (seconds since 1Jan1904=w423:timestamp)
      n149 = Format Date/Time String(time format string (%c)="%H:%M", seconds (now)=w421) -> (date/time string=w418:string)  [unwired: 1 in]
      n150 = Format Date/Time String(time format string (%c)="%d-%b-%Y", seconds (now)=w423) -> (date/time string=w419:string)  [unwired: 1 in]
      n151 = Select(t="Pass", s=w428, f="Fail") -> (s? t:f=w425:string)
      n152 = Bundle By Name(cluster=T26 {"MSPartName"="", "MSDate"="", "MSTime"="", "MSMeasurementValueArray"=[], "MSResult"=""} ("MasterSampleInfo"), "MSDate"=w419, "MSTime"=w418, "MSMeasurementValueArray"=w424, "MSResult"=w425, "MSPartName"=w417) -> (w429:T26)
      n153 = call "Send MasterSample Info_DL.vi"("error in (no error)"=w433, "MasterSampleInfo"=w429, "Message Enqueuer"=w434) -> ("error out"=w432:errorcluster)  [unwired: 7 in, 1 out]
    }
  }
  "error out" <- w10
  "SM Private Data out" <- "SM Private Data in"
